vi "Day 11 -Monkey in the Middle.vi"() -> ()   [LabVIEW 2020, in "AoC 2022.lvlib"]
uses:
  AoC 2022.lvlib
panel:
  in  "Puzzle Input":string="Monkey 0:\n  Starting items: 79, 98\n  Operation: new = old * 19\n  Test: divisible by 23\n    If true: throw to monkey 2\n    If false: throw to monkey 3\n\nMonkey 1:\n  Starting items: 54, 65, 75, 74\n  Operation: new = old + 6\n  Test: divisible by 19\n    If true: throw to monkey 2\n    If false: throw to monkey 0\n\nMonkey 2:\n  Starting items: 79, 60, 97\n  Operation: new = old * old\n  Test: divisible by 13\n    If true: throw to monkey 1\n    If false: throw to monkey 3\n\nMonkey 3:\n  Starting items: 74\n  Operation: new = old + 3\n  Test: divisible by 17\n    If true: throw to monkey 0\n    If false: throw to monkey 1"
  out "Puzzle Part-2 Answer":string
  out "Puzzle Answer":string
  # "Press Ctrl+M & Enter the Puzzle Input and run the VI"
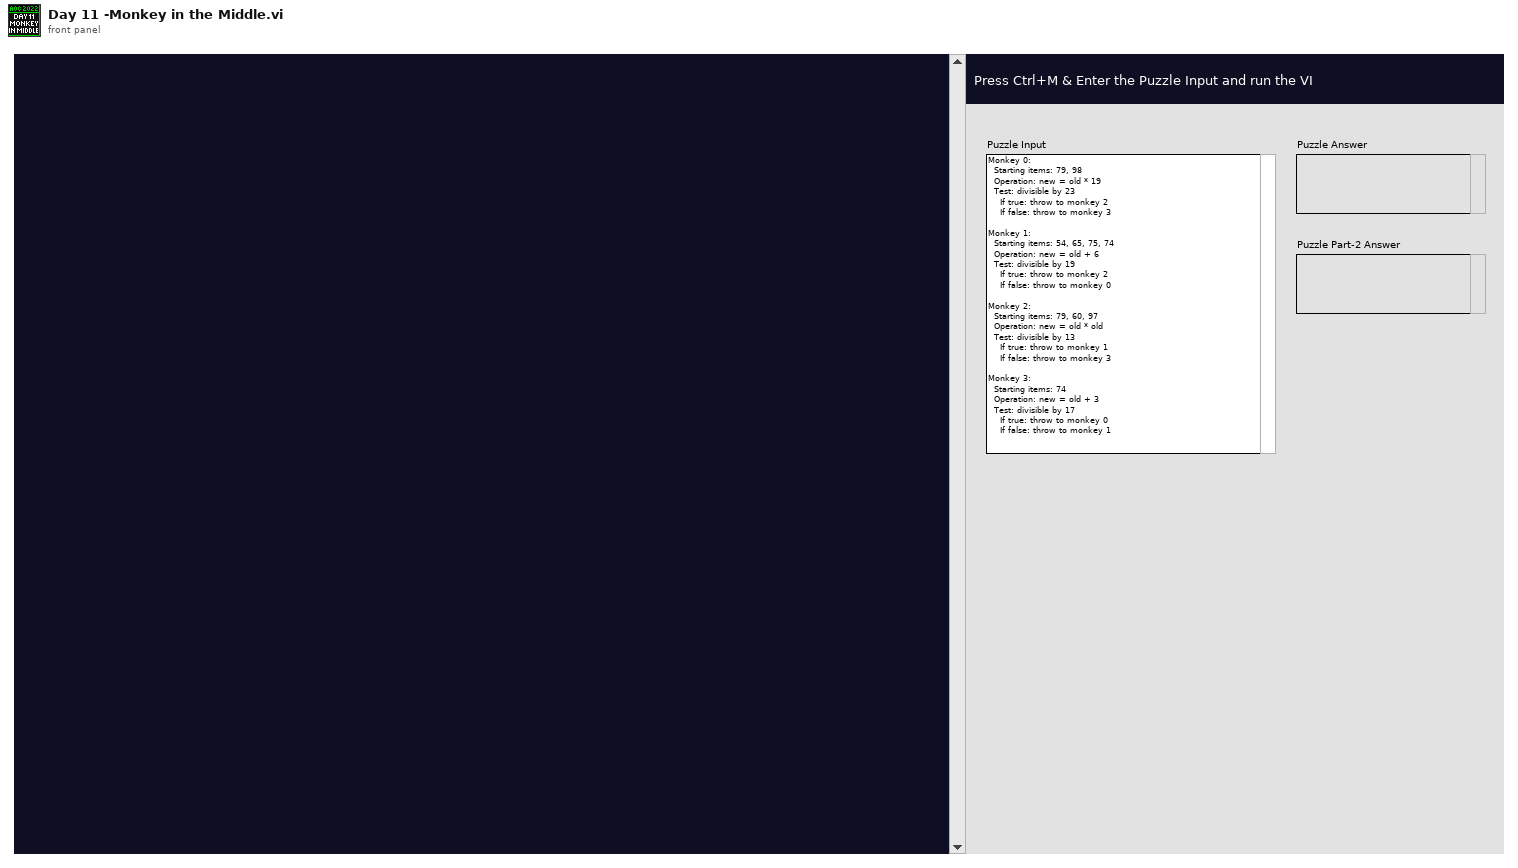
[diagram p1: front panel]
types:
  T1 = typedef "AoC 2022.lvlib/Monkeys.ctl" = map{i32, T2}
  T2 = typedef "AoC 2022.lvlib/Monkey.ctl" = cluster{"Items":u64[], "Bored Operation":string, "Inspection Operation":string, "Test: Divisible By":u64, "Test: True - Monkey":i32, "Test: False - Monkey":i32, "#Inspected":i32}
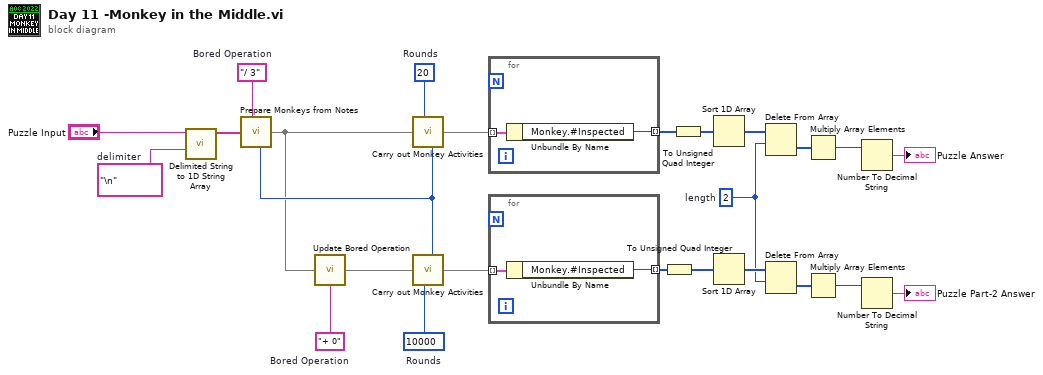
[diagram p0: block diagram]
diagram:
  w1 = "+ 0"  # Bored Operation
  w14 = 10000  # Rounds
  w16 = "/ 3"  # Bored Operation
  w7 = 2  # length
  w22 = 20  # Rounds
  w23 = "\n"  # delimiter
  n1 = call <vilib>:"Delimited String to 1D String Array.vi"("delimiter"=w23, "delimited string"="Puzzle Input") -> ("string array"=w15:string[])  [unwired: 9 in]
  n2 = call "Prepare Monkeys from Notes.vi"("Monkey Business Notes"=w15, "Bored Operation"=w16) -> ("LCD"=w6:u64, "Monkeys"=w3:T1)
  n3 = call "Update Bored Operation.vi"("Monkeys in"=w3, "Bored Operation"=w1) -> ("Monkeys out"=w2:T1)
  n4 = call "Carry out Monkey Activities.vi"("Monkeys in"=w3, "#Rounds"=w22, "LCD"=w6) -> ("Monkeys out"=w21:T1)
  n5 = call "Carry out Monkey Activities.vi"("Monkeys in"=w2, "#Rounds"=w14, "LCD"=w6) -> ("Monkeys out"=w9:T1)
  n6 = for {
    tunnel: w21 -> [w27] mode=indexing
    tunnel: [w26] -> w20 mode=indexing
    n7 = Unbundle By Name(w27) -> ("Monkey.#Inspected"=w26:i32)
  }
  n8 = for {
    tunnel: w9 -> [w29] mode=indexing
    tunnel: [w28] -> w10 mode=indexing
    n9 = Unbundle By Name(w29) -> ("Monkey.#Inspected"=w28:i32)
  }
  n10 = To Unsigned Quad Integer(1:w10) -> (0:w5:u64[])
  n11 = To Unsigned Quad Integer(1:w20) -> (0:w4:u64[])
  n12 = Sort 1D Array(array=w4) -> (sorted array=w19:u64[])
  n13 = Sort 1D Array(array=w5) -> (sorted array=w11:u64[])
  n14 = Delete From Array(array=w19, length=w7) -> (deleted portion=w18:u64[])  [unwired: 1 in, 1 out]
  n15 = Delete From Array(array=w11, length=w7) -> (deleted portion=w12:u64[])  [unwired: 1 in, 1 out]
  n16 = Multiply Array Elements(1:w18) -> (0:w17:u64)
  n17 = Multiply Array Elements(1:w12) -> (0:w13:u64)
  n18 = Number To Decimal String(number=w17) -> (decimal integer string=→"Puzzle Answer":string)  [unwired: 1 in]
  n19 = Number To Decimal String(number=w13) -> (decimal integer string=→"Puzzle Part-2 Answer":string)  [unwired: 1 in]
